vi "TickFGV.vi"(11 "Énum":enum16{"start", "tick", "get"}(ring)=enum."tick") -> (3 "timer value (s)":u32)   [LabVIEW 2020]
panel:
  # "SINGLETON FGV"
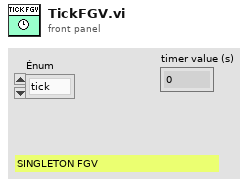
[diagram p1: front panel]
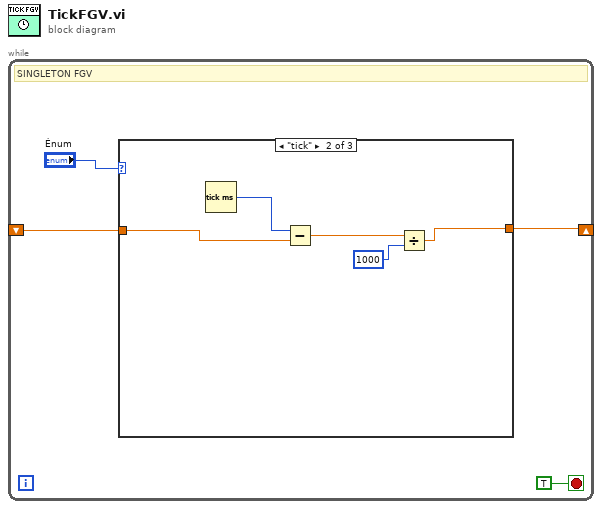
[diagram p0: block diagram]
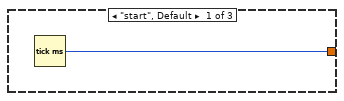
[diagram p2: hidden frame]
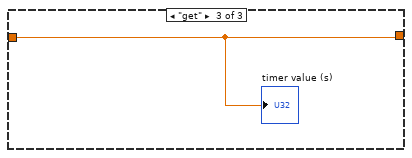
[diagram p3: hidden frame]
diagram:
  n1 = while {
    shift-right: [w2] -> _
    shift-left: _ -> [w1]
    stop <- TRUE stop-if-true
    # "SINGLETON FGV"
    n2 = case shown="\"tick\"" "Énum" {
      tunnel: [w5 w6 w11] -> w2
      tunnel: w1 -> [_ w9 w11]
      frame "start", Default {
        n3 = Tick Count (ms)() -> (millisecond timer value=w5:u32)
      }
      frame "tick" {
        n4 = Tick Count (ms)() -> (millisecond timer value=w10:u32)
        n5 = Subtract(x=w10, y=w9) -> (x-y=w8:dbl)
        n6 = Divide(x=w8, y=u32 1000) -> (x/y=w6:dbl)
      }
      frame "get" {
        "timer value (s)" <- w11
      }
    }
  }
